vi "Get Buffer.vi"(8 "error in":errorcluster, 11 "BufferWrites1SamDBL in":refnum<class "BufferWrites1SamDBL.lvclass">) -> (0 "error out":errorcluster, 2 "Buffer":dbl[](array[numeric]), 3 "BufferWrites1SamDBL out":refnum<class "BufferWrites1SamDBL.lvclass">)   [LabVIEW 2023, in "BufferWrites1SamDBL.lvclass"]
uses:
  BufferWrites1SamDBL.lvclass
  BufferWrites1SamDBL.lvclass/BufferWrites1SamDBL.ctl
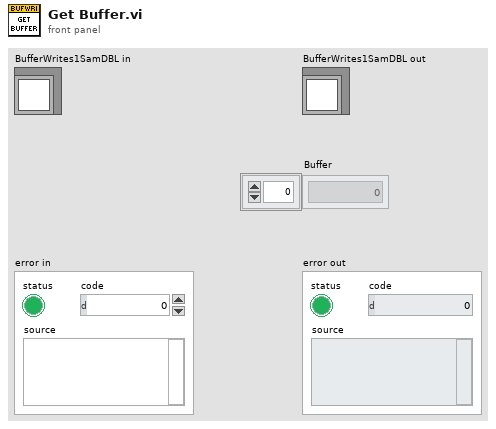
[diagram p1: front panel]
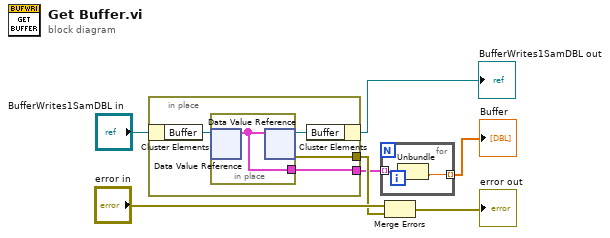
[diagram p0: block diagram]
diagram:
  n1 = in-place {
    in-place-border: [w10] -> w3
    in-place-border: [w8] -> w4
    n2 = in-place-cluster #1("BufferWrites1SamDBL in") -> ("Buffer"=w11:refnum<data-value>)
    n3 = in-place {
      in-place-border: [w12] -> w10
      n4 = in-place-dvr #2(w11) -> (w12:cluster{"Ident":string, "Value":dbl}[])  [unwired: 1 out]
      n5 = in-place-dvr #2(w12) -> (w9:refnum<data-value>, w8:errorcluster)
    }
    n6 = in-place-cluster #1("Buffer"=w9) -> (→"BufferWrites1SamDBL out":refnum<class "BufferWrites1SamDBL.lvclass">)
  }
  n7 = for {
    tunnel: w3 -> [w14] mode=indexing
    tunnel: [w13] -> w1 mode=indexing
    n8 = Unbundle(w14) -> ("Value"=w13:dbl)  [unwired: 1 out]
  }
  "Buffer" <- w1
  n9 = Merge Errors("error in", w4) -> (→"error out":errorcluster)
